vi "Execute Turn.vi"(7 "Player Color":T1, 8 "error in":errorcluster, 9 "Possible Moves":bool[][](array[boolean]), 10 "Board":T3[][](array[typedef]), 11 "Diagon Alley in":refnum<class "Diagon Alley.lvclass">) -> (0 "error out":errorcluster, 2 "Choice Coordinates":T2, 3 "Diagon Alley out":refnum<class "Diagon Alley.lvclass">)   [LabVIEW 2020, in "Reversi.lvlib" / "Diagon Alley.lvclass"]
uses:
  Diagon Alley.lvclass
  Reversi/Space Ring.ctl
  Reversi/Reversi.lvclass
  Reversi/Space Coordinates.ctl
  Reversi/Turn Enum.ctl
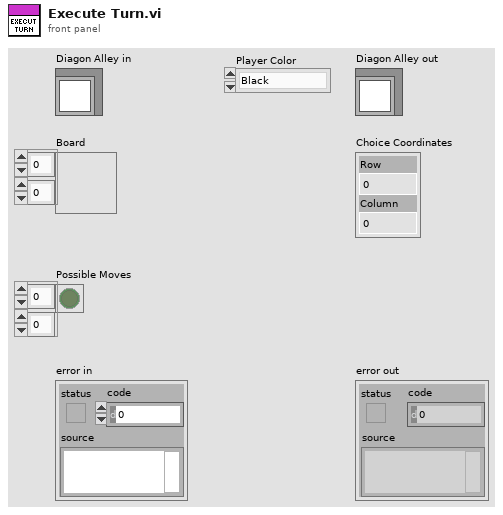
[diagram p1: front panel]
types:
  T1 = typedef "Reversi.lvlib/Reversi.lvclass/Turn Enum.ctl" = enum16{"Black", "White"}
  T2 = typedef "Reversi.lvlib/Reversi.lvclass/Space Coordinates.ctl" = cluster{"Row":i32, "Column":i32}
  T3 = typedef "Reversi.lvlib/Reversi.lvclass/Space Ring.ctl" = u16
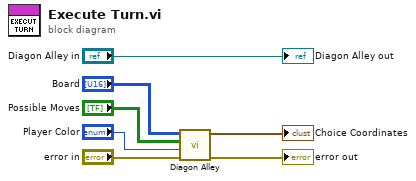
[diagram p0: block diagram]
diagram:
  n1 = call "Diagon Alley.vi"("error in"="error in", "Player Color"="Player Color", "Possible Moves"="Possible Moves", "Board"="Board") -> ("error out"=→"error out":errorcluster, "Choice Coordinates"=→"Choice Coordinates":T2)  [unwired: 6 in]
  "Diagon Alley out" <- "Diagon Alley in"
